vi "Load Panel.vi"(8 "error in (no error)":errorcluster, 10 "vi reference":refnum<vi>, 11 "value":cluster{i32[][], string[]}) -> (0 "error out":errorcluster)   [LabVIEW 2017]
panel:
  out "number of controls":i32
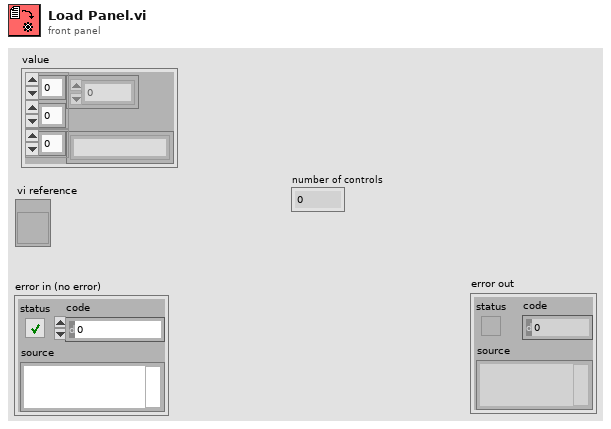
[diagram p1: front panel]
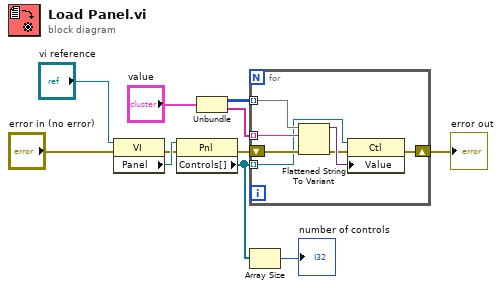
[diagram p0: block diagram]
diagram:
  n1 = property class="VI"(reference="vi reference", error in="error in (no error)") -> (error out=w8:errorcluster, "Panel"=w10:refnum<vi>)  [unwired: 1 out]
  n2 = property class="Pnl"(reference=w10, error in=w8) -> (error out=w3:errorcluster, "Controls[]"=w2:refnum<vi>[])  [unwired: 1 out]
  n3 = Unbundle("value") -> (w6:i32[][], w5:string[])
  n4 = for {
    tunnel: w2 -> [w12] mode=indexing
    shift-right: [w13] -> w7
    shift-left: w3 -> [w15]
    tunnel: w6 -> [w18] mode=indexing
    tunnel: w5 -> [w17] mode=indexing
    n5 = Flattened String To Variant(4:w15, 6:w17, 7:w18) -> (0:w14:errorcluster, 3:w16:variant)
    n6 = property class="Ctl"(reference=w12, error in=w14, "Value"=w16) -> (error out=w13:errorcluster)  [unwired: 1 out]
  }
  "error out" <- w7
  n7 = Array Size(array=w2) -> (size(s)=→"number of controls":i32)
